vi "main.vi"() -> ()   [LabVIEW 2025]
uses:
  9a674b0b-287d-4e54-8c99-c9b59376f716.vi
  System.Speech
panel:
  in  "枚举":enum16{"语音", "人脸", "手动"}(ring)
  in  "灯开关":bool
  out "布尔 2":bool
  out "回复":string
  out "布尔":bool
  in  "phrases":string[](array[string])=["你好", "打开手动模式", "很高兴见到你", "再见", "打开灯", "关闭灯", "加油小林哥", "滚吧", "打开子程序", "关闭子程序", "我饿了", "我想听歌"]
  in  "识别结果":string
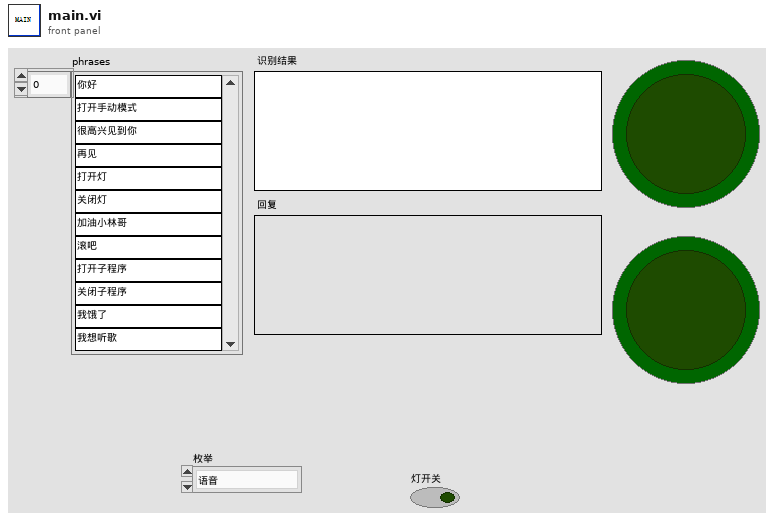
[diagram p1: front panel]
types:
  T1 = enum32{"Invalid", "Standard", "Closed", "Hidden", "Minimized", "Maximized"}
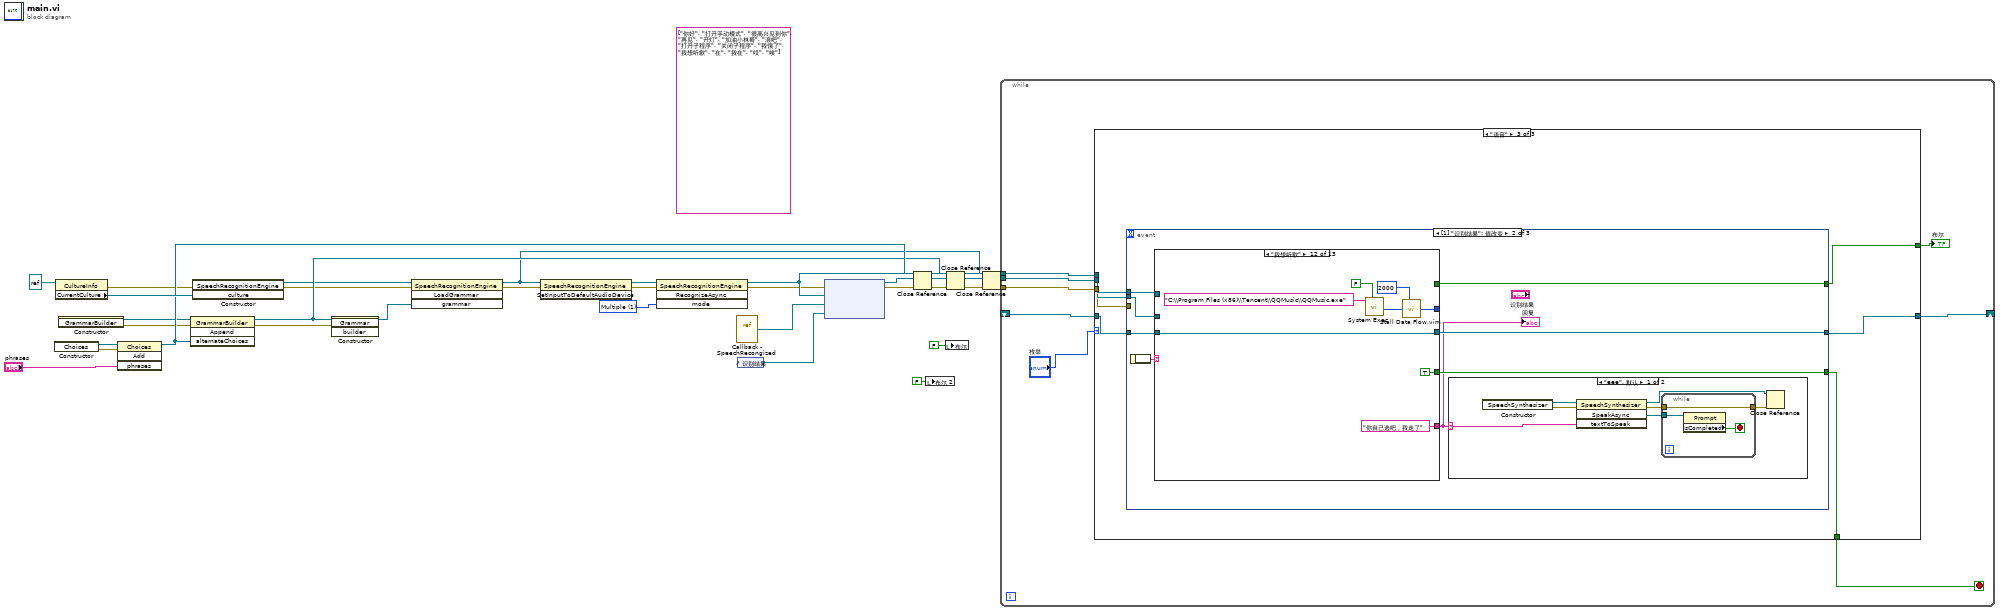
[diagram p0: block diagram]
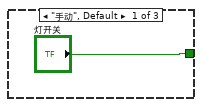
[diagram p2: hidden frame]
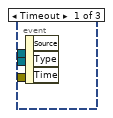
[diagram p4: hidden frame]
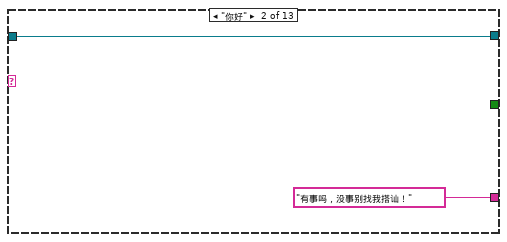
[diagram p6: hidden frame]
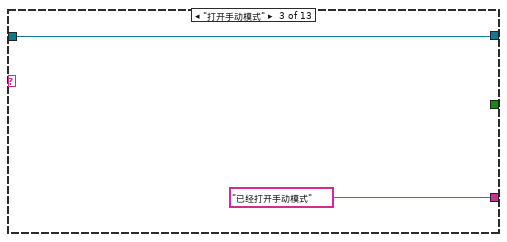
[diagram p7: hidden frame]
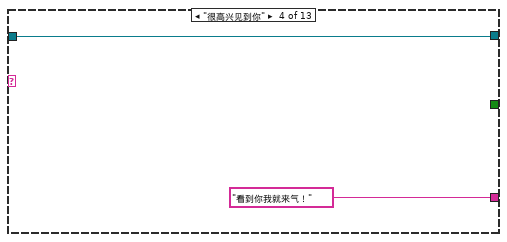
[diagram p8: hidden frame]
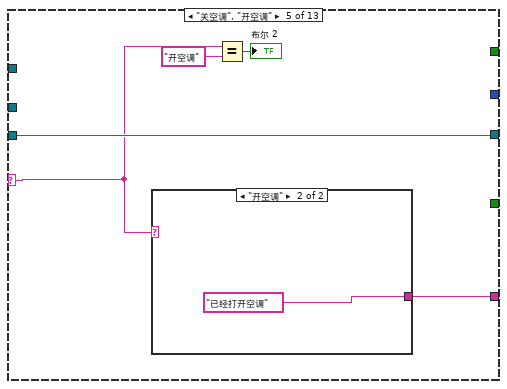
[diagram p9: hidden frame]
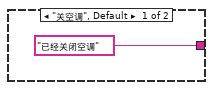
[diagram p10: hidden frame]
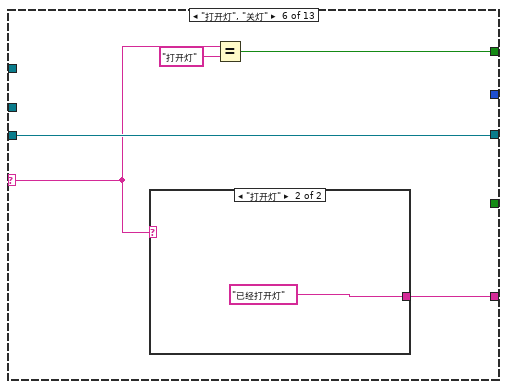
[diagram p11: hidden frame]
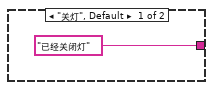
[diagram p12: hidden frame]
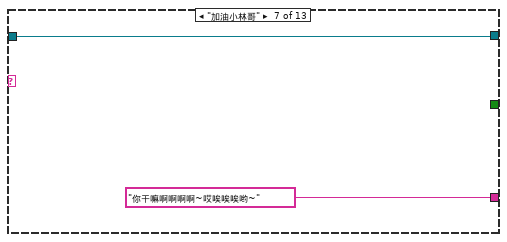
[diagram p13: hidden frame]
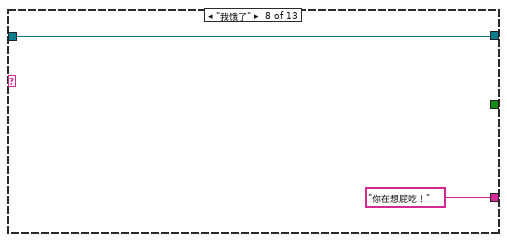
[diagram p14: hidden frame]
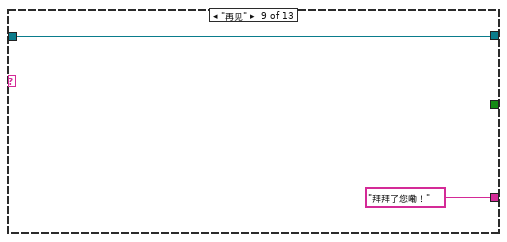
[diagram p15: hidden frame]
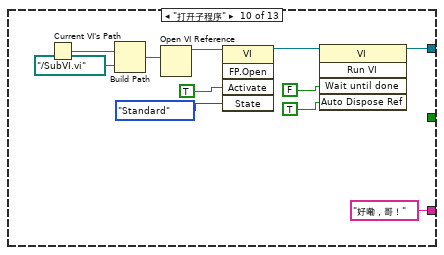
[diagram p16: hidden frame]
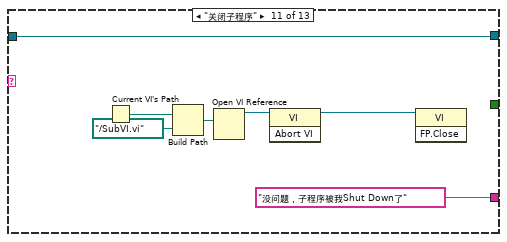
[diagram p17: hidden frame]
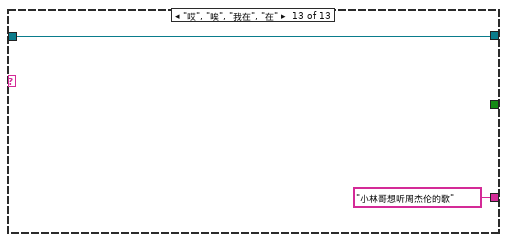
[diagram p18: hidden frame]
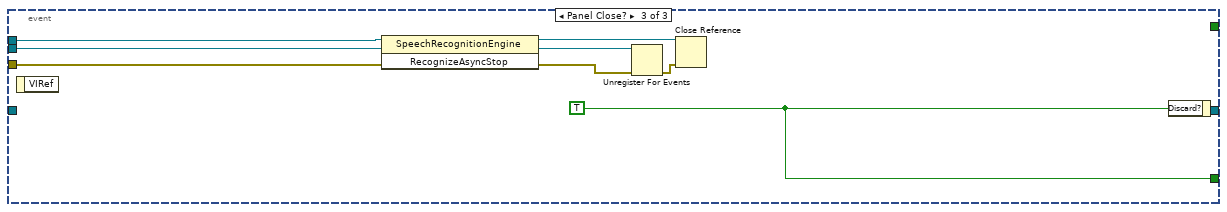
[diagram p20: hidden frame]
diagram:
  (unwired) string[] ["你好", "打开手动模式", "很高兴见到你", "再见", "开灯", "加油小林哥", "滚吧", "打开子程序", "关闭子程序", "我饿了", "我想听歌", "在", "我在", "哎", "唉"] ("phrases")
  w11 = 1 items=["Single", "Multiple"] ("mode")
  n1 = constructor class="Choices"() -> (reference out=w4:refnum<k24>, error out=w6:errorcluster)  [unwired: 3 in, 1 out]
  n2 = property class="CultureInfo"(reference=refnum<k24> refnum ("引用")) -> (error out=w15:errorcluster, "CurrentCulture"=w25:refnum<k24>)  [unwired: 1 in, 1 out]
  n3 = constructor class="GrammarBuilder"() -> (reference out=w5:refnum<k24>, error out=w7:errorcluster)  [unwired: 3 in, 1 out]
  n4 = invoke class="Choices" method="Add"(reference=w4, error in=w6, "phrases"="phrases") -> (reference out=w24:refnum<k24>)  [unwired: 1 in, 3 out]
  n5 = invoke class="GrammarBuilder" method="Append"(reference=w5, error in=w7, "alternateChoices"=w24) -> (reference out=w23:refnum<k24>, error out=w16:errorcluster)  [unwired: 1 in, 2 out]
  n6 = constructor class="SpeechRecognitionEngine"(error in=w15, "culture"=w25) -> (reference out=w8:refnum<k24>, error out=w12:errorcluster)  [unwired: 2 in, 2 out]
  n7 = constructor class="Grammar"(error in=w16, "builder"=w23) -> (reference out=w9:refnum<k24>)  [unwired: 2 in, 3 out]
  n8 = invoke class="SpeechRecognitionEngine" method="LoadGrammar"(reference=w8, error in=w12, "grammar"=w9) -> (reference out=w22:refnum<k24>, error out=w17:errorcluster)  [unwired: 1 in, 2 out]
  n9 = invoke class="SpeechRecognitionEngine" method="SetInputToDefaultAudioDevice"(reference=w22, error in=w17) -> (reference out=w10:refnum<k24>, error out=w13:errorcluster)  [unwired: 1 in, 1 out]
  n10 = invoke class="SpeechRecognitionEngine" method="RecognizeAsync"(reference=w10, error in=w13, "mode"=w11) -> (reference out=w28:refnum<k24>, error out=w18:errorcluster)  [unwired: 1 in, 2 out]
  n11 = vi-ref "Callback - SpeechRecongized.vi"() -> (w14:refnum<vi>)
  n12 = control-ref of="识别结果"() -> (w29:refnum<vi>)
  n13 = node(w18, w28, w14, w29) -> (w27:refnum<k27>, w19:errorcluster)  [unwired: 1 in]
  n14 = Close Reference(reference=w24, error in (no error)=w19) -> (error out=w20:errorcluster)
  n15 = local write "布尔 2"(FALSE ("布尔")) -> ()
  n16 = local write "布尔"(FALSE ("布尔")) -> ()
  n17 = Close Reference(reference=w23, error in (no error)=w20) -> (error out=w21:errorcluster)
  n18 = Close Reference(reference=w22, error in (no error)=w21) -> (error out=w30:errorcluster)
  n19 = while {
    tunnel: w30 -> [w35]
    tunnel: w28 -> [w37]
    tunnel: w27 -> [w36]
    shift-right: [w34] -> _
    shift-left: _ -> [w33]
    stop <- w38 stop-if-true
    n20 = case shown="\"语音\"" "枚举" {
      tunnel: [_ _ w46] -> w38
      tunnel: w37 -> [_ _ w45]
      tunnel: w36 -> [_ _ w44]
      tunnel: w35 -> [_ _ w43]
      tunnel: [_ _ w42] -> w34
      tunnel: w33 -> [_ _ w41]
      tunnel: ["灯开关" _ w40] -> w32
      frame "手动", Default {
      }
      frame "人脸" {
      }
      frame "语音" {
        n21 = event shown="[1] \"识别结果\": 值改变" {
          selector: _ -> [_ _ _]
          dyn-events: _ -> [_ _ _]
          timeout: _ -> [_ _ _]
          tunnel: [_ w49 w125] -> w46
          tunnel: w45 -> [_ w53 w121]
          tunnel: w44 -> [_ w52 w124]
          tunnel: w43 -> [_ _ w122]
          tunnel: [_ w51 _] -> w42
          tunnel: w41 -> [_ w50 _]
          tunnel: [_ w47 _] -> w40
          event Timeout {
            n22 = event-data() -> ()  [unwired: 1 in, 3 out]
          }
          event "识别结果": Value Change {
            n23 = event-data() -> ("NewVal"=w54:string)  [unwired: 1 in]
            n24 = case shown="\"我想听歌\"" w54 {
              selector: w54 -> [_ _ _ _ w63 w71 _ _ _ _ _ _ _]
              tunnel: w53 -> [_ _ _ _ _ _ _ _ _ _ _ _ _]
              tunnel: w52 -> [_ _ _ _ _ _ _ _ _ _ _ _ _]
              tunnel: [w55 w57 w59 w61 w66 w73 w77 w79 w81 w84 w96 w107 w109] -> w51
              tunnel: w50 -> [w55 w57 w59 w61 w66 w73 w77 w79 w81 _ w96 w107 w109]
              tunnel: [_ "有事吗，没事别找我搭讪！" ("textToSpeak") "已经打开手动模式" ("textToSpeak") "看到你我就来气！" ("textToSpeak") w62 w70 "你干嘛啊啊啊啊~哎唉唉唉哟~" ("textToSpeak") "你在想屁吃！" ("textToSpeak") "拜拜了您嘞！" ("textToSpeak") "好嘞，哥！" ("textToSpeak") "没问题，子程序被我Shut Down了" ("textToSpeak") "你自己选吧，我走了" ("textToSpeak") "小林哥想听周杰伦的歌" ("textToSpeak")] -> w48
              tunnel: [_ _ _ _ _ _ _ _ _ _ _ TRUE _] -> w49
              tunnel: [_ _ _ _ _ _ _ _ _ _ _ w101 _] -> _
              tunnel: [_ _ _ _ _ w69 _ _ _ _ _ _ _] -> w47
              frame "eee", Default {
              }
              frame "你好" {
              }
              frame "打开手动模式" {
              }
              frame "很高兴见到你" {
              }
              frame "关空调", "开空调" {
                n25 = case shown="\"开空调\"" w63 {
                  tunnel: ["已经关闭空调" "已经打开空调"] -> w62
                  frame "关空调", Default {
                  }
                  frame "开空调" {
                  }
                }
                n26 = Equal?(x=w63, y="开空调") -> (x = y?=→"布尔 2":bool)
              }
              frame "打开灯", "关灯" {
                n27 = case shown="\"打开灯\"" w71 {
                  tunnel: ["已经关闭灯" "已经打开灯"] -> w70
                  frame "关灯", Default {
                  }
                  frame "打开灯" {
                  }
                }
                n28 = Equal?(x=w71, y="打开灯") -> (x = y?=w69:bool)
              }
              frame "加油小林哥" {
              }
              frame "我饿了" {
              }
              frame "再见" {
              }
              frame "打开子程序" {
                n29 = Current VI's Path() -> (path=w89:path)
                n30 = Build Path(base path=w89, name or relative path=path "../SubVI.vi" ("名称或相对路径")) -> (appended path=w87:path)
                n31 = Open VI Reference(vi path=w87) -> (vi reference=w92:refnum<vi>)  [unwired: 5 in, 1 out]
                n32 = invoke class="VI" method="FP.Open"(reference=w92, "Activate"=TRUE ("激活？"), "State"=T1."Standard" ("状态")) -> (reference out=w85:refnum<vi>)  [unwired: 2 in, 4 out]
                n33 = invoke class="VI" method="Run VI"(reference=w85, "Wait until done"=FALSE ("结束前等待"), "Auto Dispose Ref"=TRUE ("自动销毁引用")) -> (reference out=w84:refnum<vi>)  [unwired: 2 in, 4 out]
              }
              frame "关闭子程序" {
                n34 = Current VI's Path() -> (path=w99:path)
                n35 = Build Path(base path=w99, name or relative path=path "../SubVI.vi" ("名称或相对路径")) -> (appended path=w97:path)
                n36 = Open VI Reference(vi path=w97) -> (vi reference=w94:refnum<vi>)  [unwired: 5 in, 1 out]
                n37 = invoke class="VI" method="Abort VI"(reference=w94) -> (reference out=w93:refnum<vi>)  [unwired: 2 in, 2 out]
                n38 = invoke class="VI" method="FP.Close"(reference=w93) -> ()  [unwired: 2 in, 3 out]
              }
              frame "我想听歌" {
                n39 = call <vilib>:"System Exec.vi"("wait until completion? (T)"=FALSE, "command line"="C:\\Program Files (x86)\\Tencent\\QQMusic\\QQMusic.exe") -> ("return code"=w103:i32)  [unwired: 6 in, 3 out]
                n40 = call "Stall Data Flow.vim"("value in"=w103, "milliseconds to wait"=u32 2000) -> ("value out"=w101:i32)  [unwired: 1 out]
              }
              frame "哎", "唉", "我在", "在" {
              }
            }
            "回复" <- w48
            n41 = case shown="\"eee\", 默认" w48 {
              selector: w48 -> [w110 _]
              frame "eee", Default {
                n42 = constructor class="SpeechSynthesizer"() -> (reference out=w116:refnum<k24>, error out=w115:errorcluster)  [unwired: 3 in, 1 out]
                n43 = invoke class="SpeechSynthesizer" method="SpeakAsync"(reference=w116, error in=w115, "textToSpeak"=w110) -> (reference out=w113:refnum<k24>, error out=w111:errorcluster, "SpeakAsync"=w114:refnum<k24>)  [unwired: 1 in, 1 out]
                n44 = while {
                  tunnel: w114 -> [w119]
                  tunnel: [w117] -> w112
                  tunnel: w111 -> [w117]
                  stop <- w118 stop-if-true
                  n45 = property on="属性节点" class="Prompt"(reference=w119) -> ("IsCompleted"=w118:bool)  [unwired: 1 in, 2 out]
                }
                n46 = Close Reference(reference=w113, error in (no error)=w112) -> ()  [unwired: 1 out]
              }
              frame "" {
              }
            }
          }
          event Panel Close? {
            w125 = TRUE ("放弃？")
            n47 = event-data() -> ()  [unwired: 1 in, 1 out]
            n48 = invoke class="SpeechRecognitionEngine" method="RecognizeAsyncStop"(reference=w121) -> (reference out=w120:refnum<k24>)  [unwired: 2 in, 2 out]
            n49 = Unregister For Events(event registration refnum=w124, error in=w122) -> (error out=w123:errorcluster)
            n50 = Close Reference(reference=w120, error in (no error)=w123) -> ()  [unwired: 1 out]
            n51 = event-data("Discard?"=w125) -> ()  [unwired: 1 in, 1 out]
          }
        }
      }
    }
    "布尔" <- w32
  }
